vi "ReadBuffers.vi"(7 "CheckCap":bool, 8 "error in (no error)":errorcluster, 9 "Status":refnum<vi>, 10 "VISA resource name in":refnum<visa-resource-name>, 11 "XYGraph in":refnum<vi>) -> (0 "error out":errorcluster, 1 "Cluster":T2, 2 "Array":dbl[][](array[numeric]), 3 "VISA Refnum out":refnum<visa-resource-name>, 4 "CapacitanceRecords":T1[](array[typedef]))   [LabVIEW 2020]
uses:
  CapacitanceRecord.ctl
  Keithley 2600 Series/Keithley 2600 Series.lvlib
panel:
  out "error out 2":errorcluster
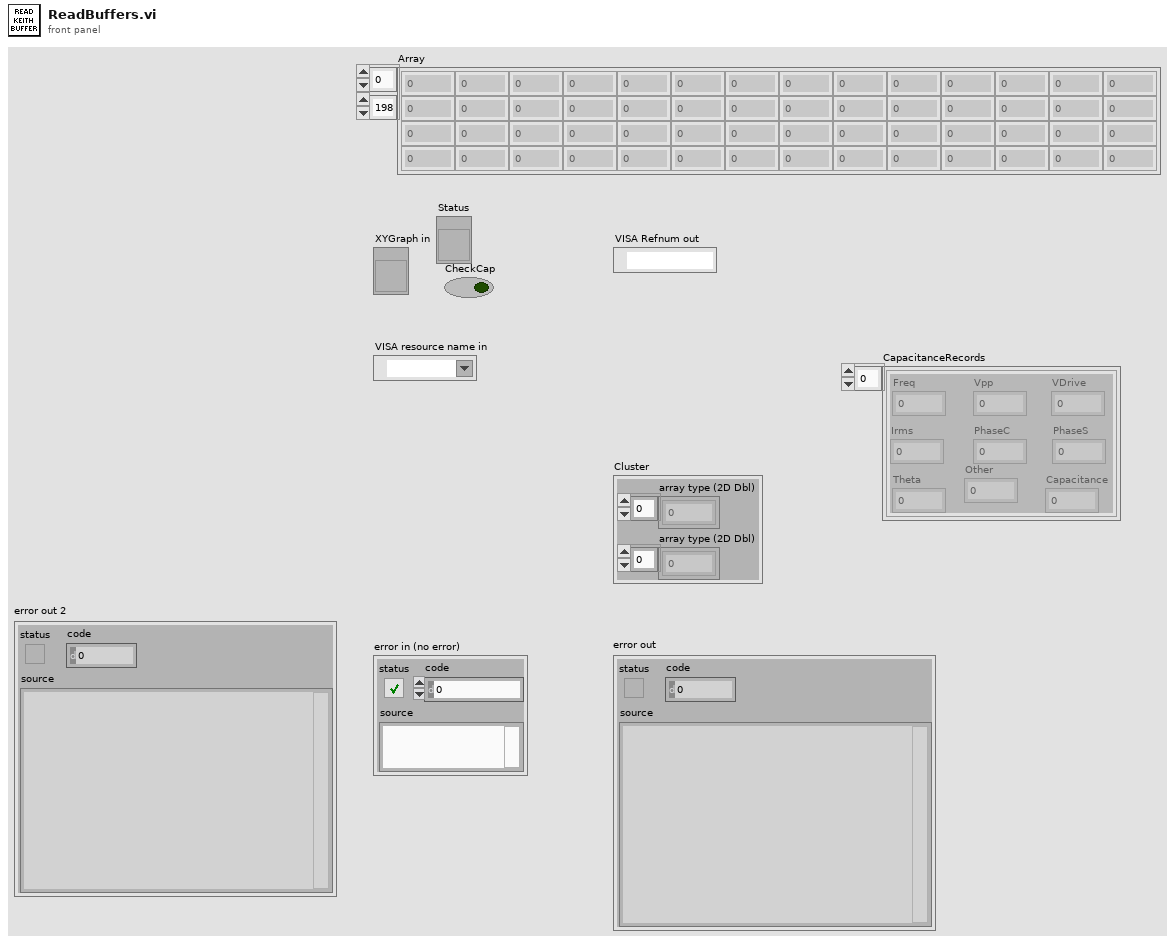
[diagram p1: front panel]
types:
  T1 = typedef "CapacitanceRecord.ctl" = cluster{"Freq":dbl, "Vpp":dbl, "PhaseS":dbl, "Irms":dbl, "PhaseC":dbl, "Theta":dbl, "VDrive":dbl, "Capacitance":dbl, "Other":dbl}
  T2 = cluster{"array type (2D Dbl)":dbl[], "array type (2D Dbl)":dbl[]}
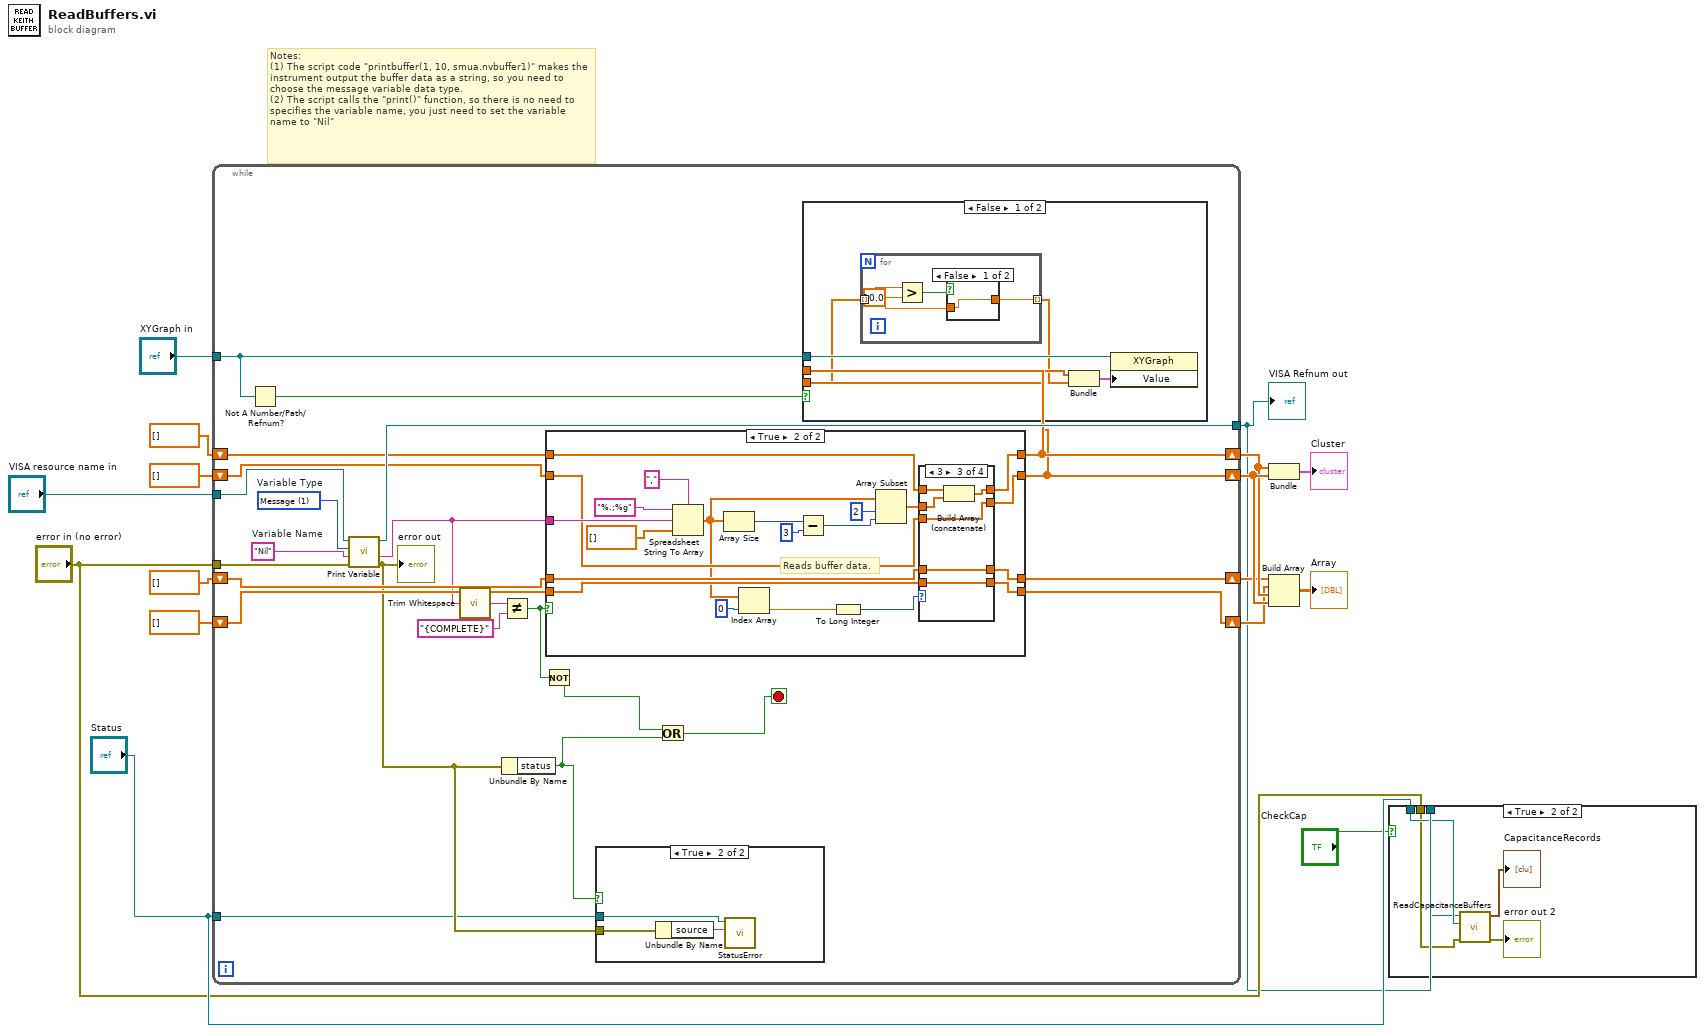
[diagram p0: block diagram]
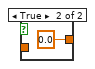
[diagram p4: hidden frame]
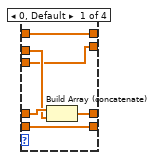
[diagram p7: hidden frame]
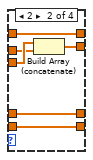
[diagram p8: hidden frame]
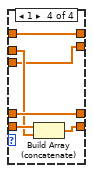
[diagram p9: hidden frame]
diagram:
  # "Notes: \n(1) The script code \"printbuffer(1, 10, smua.nvbuffer1)\" makes the instrument output the buffer data as a string, so you need to choose the message variable data type.\n(2) The script calls the \"print()\" function, so there is no need to specifies the variable name, you just need to set the variable name to \"Nil\""
  n1 = while {
    tunnel: "VISA resource name in" -> [w38]
    tunnel: "error in (no error)" -> [w37]
    tunnel: [w36] -> w2
    shift-right: [w31] -> w12
    shift-left: dbl[] [] ("array type (2D Dbl)") -> [w32]
    shift-right: [w24] -> w14
    shift-left: dbl[] [] ("array type (2D Dbl)") -> [w30]
    shift-right: [w35] -> w11
    shift-left: dbl[] [] ("array type (2D Dbl)") -> [w34]
    shift-right: [w23] -> w15
    shift-left: dbl[] [] ("array type (2D Dbl)") -> [w33]
    tunnel: "XYGraph in" -> [w26]
    tunnel: "Status" -> [w18]
    stop <- w21 stop-if-true
    w40 = 1 items=["Number", "Message"]  # Variable Type
    w39 = "Nil"  # Variable Name
    n2 = Not A Number/Path/Refnum?(number/path/refnum=w26) -> (NaN/Path/Refnum?=w25:bool)
    n3 = call "Print Variable.vi"("error in (no error)"=w37, "Variable Name"=w39, "Variable Type (0: Number)"=w40, "VISA resource name"=w38) -> ("error out"=w20:errorcluster, "Message"=w17:string, "VISA resource name out"=w36:refnum<visa-resource-name>)  [unwired: 4 in, 1 out]
    "error out" <- w20
    n4 = call <vilib>:"Trim Whitespace.vi"("string"=w17) -> ("trimmed string"=w29:string)  [unwired: 1 in]
    n5 = Not Equal?(x=w29, y="{COMPLETE}") -> (x != y?=w27:bool)
    n6 = Unbundle By Name(w20) -> ("status"=w19:bool)
    n7 = Not(x=w27) -> (.not. x?=w22:bool)
    n8 = case shown="True" w27 {
      tunnel: w17 -> [_ w76]
      tunnel: [w58 w74] -> w35
      tunnel: w34 -> [w58 w73]
      tunnel: [w56 w71] -> w23
      tunnel: w33 -> [w56 w69]
      tunnel: w32 -> [w57 w68]
      tunnel: [w57 w67] -> w31
      tunnel: w30 -> [w55 w66]
      tunnel: [w55 w65] -> w24
      frame False {
      }
      frame True {
        # "Reads buffer data."
        n9 = Spreadsheet String To Array(delimiter (Tab)=",", format string="%.;%g", spreadsheet string=w76, array type (2D Dbl)=dbl[] []) -> (array=w62:dbl[])
        n10 = Array Size(array=w62) -> (size(s)=w61:i32)
        n11 = Index Array(array=w62, index=0) -> (element=w72:dbl)
        n12 = Subtract(x=w61, y=3) -> (x-y=w59:i32)
        n13 = To Long Integer(number=w72) -> (32bit integer=w70:i32)
        n14 = Array Subset(array=w62, index=2, length=w59) -> (w64:dbl[])
        n15 = case shown="3" w70 {
          tunnel: [w83 w91 w97 w103] -> w74
          tunnel: w73 -> [w85 w91 w97 w103]
          tunnel: [w82 w86 w96 w99] -> w71
          tunnel: w64 -> [w84 w89 w93 w101]
          tunnel: w69 -> [w82 w90 w96 w99]
          tunnel: w68 -> [w81 w88 w95 w102]
          tunnel: [w81 w88 w95 w100] -> w67
          tunnel: w66 -> [w80 w87 w94 w98]
          tunnel: [w80 w87 w92 w98] -> w65
          frame 0, Default {
            n16 = Build Array (concatenate)(w85, w84) -> (w83:dbl[])
          }
          frame 2 {
            n17 = Build Array (concatenate)(w90, w89) -> (w86:dbl[])
          }
          frame 3 {
            n18 = Build Array (concatenate)(w94, w93) -> (w92:dbl[])
          }
          frame 1 {
            n19 = Build Array (concatenate)(w102, w101) -> (w100:dbl[])
          }
        }
      }
    }
    n20 = case shown="True" w19 {
      tunnel: w20 -> [_ w42]
      tunnel: w18 -> [_ w41]
      frame False {
      }
      frame True {
        n21 = Unbundle By Name(w42) -> ("source"=w43:string)
        n22 = call "StatusError.vi"("Text.Text"=w43, "String in"=w41) -> ()  [unwired: 10 in]
      }
    }
    n23 = Or(x=w22, y=w19) -> (x .or. y?=w21:bool)
    n24 = case shown="False" w25 {
      tunnel: w24 -> [w47 _]
      tunnel: w23 -> [w45 _]
      tunnel: w26 -> [w46 _]
      frame False {
        n25 = for {
          tunnel: w45 -> [w50] mode=indexing
          tunnel: [w51] -> w44 mode=indexing
          n26 = Greater?(x=w50, y=10.0) -> (0:w52:bool)
          n27 = case shown="False" w52 {
            tunnel: [w53 0.0] -> w51
            tunnel: w50 -> [w53 _]
            frame False {
            }
            frame True {
            }
          }
        }
        n28 = Bundle("array type (2D Dbl)"=w47, w44) -> (w48:cluster{"array type (2D Dbl)":dbl[], dbl[]})  [unwired: 1 in]
        n29 = property class="XYGraph"(reference=w46, "Value"=w48) -> ()  [unwired: 1 in, 2 out]
      }
      frame True {
      }
    }
  }
  "VISA Refnum out" <- w2
  n30 = Bundle("array type (2D Dbl)"=w14, "array type (2D Dbl)"=w15) -> (→"Cluster":T2)  [unwired: 1 in]
  n31 = Build Array(w11, w12, w14, w15) -> (→"Array":dbl[][])
  n32 = case shown="True" "CheckCap" {
    tunnel: "Status" -> [_ w108]
    tunnel: "error in (no error)" -> [_ w107]
    tunnel: w2 -> [_ w106]
    frame False {
    }
    frame True {
      n33 = call "ReadCapacitanceBuffers.vi"("error in (no error)"=w107, "Status"=w108, "VISA Refnum in"=w106) -> ("error out"=→"error out 2":errorcluster, "CapacitanceInfos"=→"CapacitanceRecords":T1[])  [unwired: 6 in, 1 out]
    }
  }
